vi "Automatic_FileName_sub.vi"(1 "#bin-histogram":i32, 2 "bin / ms":i32, 3 "F2 save directory":path, 4 "file path":path) -> (0 "F2 output path":path)   [LabVIEW 2009]
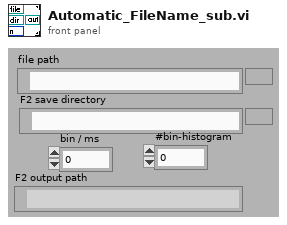
[diagram p1: front panel]
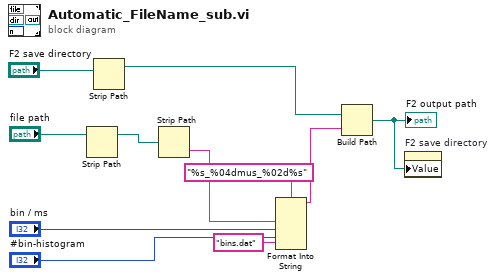
[diagram p0: block diagram]
diagram:
  n1 = Strip Path(path="file path") -> (stripped path=w10:path)  [unwired: 1 out]
  n2 = Strip Path(path="F2 save directory") -> (stripped path=w5:path)  [unwired: 1 out]
  n3 = Strip Path(path=w10) -> (name=w8:string)  [unwired: 1 out]
  n4 = Format Into String(format string="%s_%04dmus_%02d%s", w8, "bin / ms", "#bin-histogram", "bins.dat" ("input 2")) -> (resulting string=w4:string)  [unwired: 2 in, 1 out]
  n5 = Build Path(base path=w5, name or relative path=w4) -> (appended path=w3:path)
  "F2 output path" <- w3
  n6 = property on="F2 save directory" class="Path"("Value"=w3) -> ()  [unwired: 2 in, 2 out]
